vi "Read GObjectRef.vi"(8 "error in (no error)":errorcluster, 11 "GObject in":refnum<class "GObject.lvclass">) -> (0 "error out":errorcluster, 2 "ref":refnum<vi>, 3 "GObject out":refnum<class "GObject.lvclass">)   [LabVIEW 2023, in "TLC_Scripto.lvlib" / "GObject.lvclass"]
uses:
  GObject.lvclass
  C:/projects/TLC_Scripto/Source/Generic/Generic.lvclass
  Generic/Read ref.vi
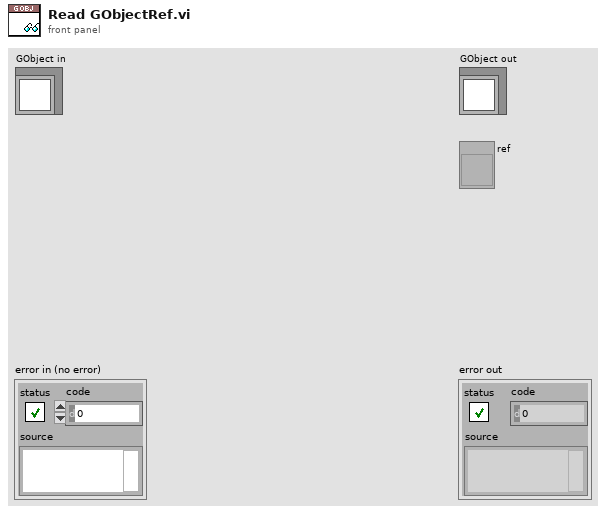
[diagram p1: front panel]
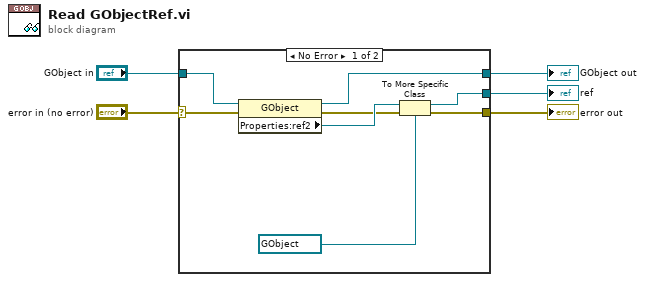
[diagram p0: block diagram]
diagram:
  n1 = case shown="No Error" "error in (no error)" {
    selector: "error in (no error)" -> [w9 w14]
    tunnel: [w8 w14] -> w4
    tunnel: [w7 w15] -> w2
    tunnel: "GObject in" -> [w6 w15]
    tunnel: [w11 _] -> w1
    frame No Error {
      n2 = property class="GObject"(reference=w6, error in=w9) -> (reference out=w7:refnum<class "GObject.lvclass">, error out=w10:errorcluster, "Properties:ref2"=w13:refnum<vi>)
      n3 = To More Specific Class(target class=refnum<vi> refnum ("ref"), reference=w13, error in=w10) -> (specific class reference=w11:refnum<vi>, error out=w8:errorcluster)
    }
    frame Error {
    }
  }
  "error out" <- w4
  "GObject out" <- w2
  "ref" <- w1
